vi "read_channel_system.vi"() -> ()   [LabVIEW 2018]
doc: "MeasGUI - Measurement Graphics User Interface\nCopyright (c) 2018 Frans Korhonen\n\nMeasGUI was originally developed at Institute for Atmospheric \nand Earth System Research / Physics, Faculty of Science, \nUniversity of Helsinki, Finland\n\nAssistance, experience and feedback from following persons have been \ncritical in development of MeasGUI: Michel Attoui, Juha Kangasluoma, \nLauri Ahonen, Ella Häkkinen, Markku Kulmala and Tuukka Petäjä.\n\nThis file is part of MeasGUI.\n\nThis Source Code Form is subject to the terms of the Mozilla Public\nLicense, v. 2.0. If a copy of the MPL was not distributed with this\nfile, You can obtain one at http://mozilla.org/MPL/2.0/."
panel:
  in  "FileName":string="\\\\.\\pipe\\cpc_out"
  in  "stop":bool
  out "string_out":string
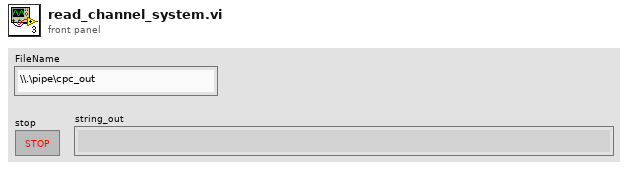
[diagram p1: front panel]
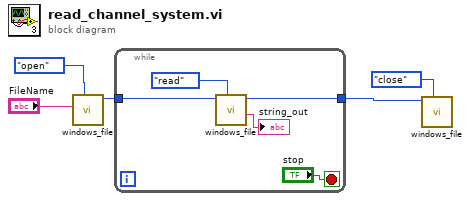
[diagram p0: block diagram]
diagram:
  n1 = call "windows_file.vi"("operation"=enum16{"open", "close", "read", "write"}."open", "FileName"="FileName") -> ("handle_out"=w3:i32)  [unwired: 8 in, 1 out]
  n2 = while {
    tunnel: w3 -> [w10]
    tunnel: [w6] -> w2
    stop <- "stop" stop-if-true
    n3 = call "windows_file.vi"("operation"=enum16{"open", "close", "read", "write"}."read", "handle_in"=w10) -> ("string_out"=→"string_out":string, "handle_out"=w6:i32)  [unwired: 8 in]
  }
  n4 = call "windows_file.vi"("operation"=enum16{"open", "close", "read", "write"}."close", "handle_in"=w2) -> ()  [unwired: 8 in, 2 out]
